vi "Start Execution Units.vi"(8 "error in (no error)":errorcluster, 11 "RT State Variables in":T1 {"Execution Unit Runtime Information"."Outgoing Data References"."Data Reference" format="%.0x"; "Execution Unit Runtime Information"."Incoming Data References" format="%.0x"}) -> (0 "error out":errorcluster, 3 "RT State Variables out":T1 {"Execution Unit Runtime Information"."Outgoing Data References"."Data Reference" format="%.0x"; "Execution Unit Runtime Information"."Incoming Data References" format="%.0x"})   [LabVIEW 2020, in "Communication Bus Template Engine.lvlib"]
uses:
  Communication Bus Template Engine.lvlib
  Includes/Communication Bus Interfaces.lvlibp/Execution Unit/Execution Unit/Execution Unit.lvclass
  <vilib>/NI/NIVS Inline Async API/_VS Inline Async API/VS Inline Async API/VS Inline Async API.lvclass
  RTStateVariables.ctl
  <vilib>/NI VeriStand/Custom Device API/Data Reference.ctl
  <vilib>/NI VeriStand/Custom Device API/Custom Device API.lvlib
  <vilib>/NI VeriStand/Custom Device API/Block Data Reference.ctl
  Execution Unit Runtime Information.ctl
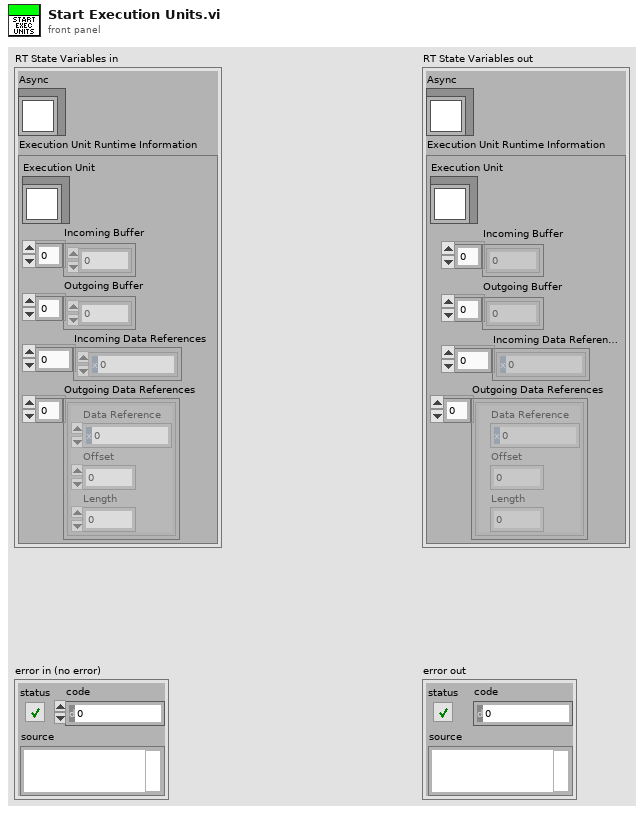
[diagram p1: front panel]
types:
  T1 = typedef "Communication Bus Template Engine.lvlib/RTStateVariables.ctl" = cluster{"Async":refnum<class "VS Inline Async API.lvclass">, "Execution Unit Runtime Information":T2}
  T2 = typedef "Communication Bus Template Engine.lvlib/Execution Unit Runtime Information.ctl" = cluster{"Execution Unit":refnum<class "Execution Unit.lvclass">, "Incoming Buffer":dbl[], "Outgoing Buffer":dbl[], "Incoming Data References":T3[], "Outgoing Data References":T4[]}
  T3 = typedef "Custom Device API.lvlib/Data Reference.ctl" = i32
  T4 = typedef "Custom Device API.lvlib/Block Data Reference.ctl" = cluster{"Data Reference":T3, "Offset":u64, "Length":u64}
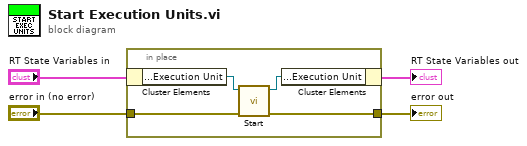
[diagram p0: block diagram]
diagram:
  n1 = in-place {
    in-place-border: "error in (no error)" -> [w6]
    in-place-border: [w5] -> w4
    n2 = in-place-cluster #1("RT State Variables in") -> ("Execution Unit Runtime Information.Execution Unit"=w8:refnum<class "Execution Unit.lvclass">)
    n3 = call-dynamic "Start.vi"("error in (no error)"=w6, "Execution Unit in"=w8) -> ("error out"=w5:errorcluster, "Execution Unit out"=w7:refnum<class "Execution Unit.lvclass">)  [unwired: 8 in]
    n4 = in-place-cluster #1("Execution Unit Runtime Information.Execution Unit"=w7) -> (→"RT State Variables out":T1)
  }
  "error out" <- w4
